vi "Config - Fire CMD.vi"(8 "error in (no error)":errorcluster, 10 "Config CMD":T1, 11 "View Model":T2) -> (0 "error out":errorcluster, 3 "View Model":T2)   [LabVIEW 2017]
doc: "Generates User Event for Configuration command."
uses:
  View Model/Controls/View Model.ctl
  Error Handler/Controls/Error Model.ctl
  Error Handler/Controls/Error Data.ctl
  Error Handler/Controls/Error Type.ctl
  View Model/Controls/Shared Model.ctl
  Controls/Config Model.ctl
  Controls/Config CMD.ctl
  Controls/Config Data.ctl
  ATM Controller/Controls/Controller Model.ctl
  ATM Controller/Controls/Controller Overhead.ctl
  ATM Controller/Controls/Controller States.ctl
  ATM Controller/Controls/Controller Message Data.ctl
  ATM Controller/Controls/Controller Message Name.ctl
  Views/User Console View/Controls/User Console - Keypad.ctl
  Views/User Console View/Controls/User Console - Transactions.ctl
  ATM Controller/Controls/Controller CMD.ctl
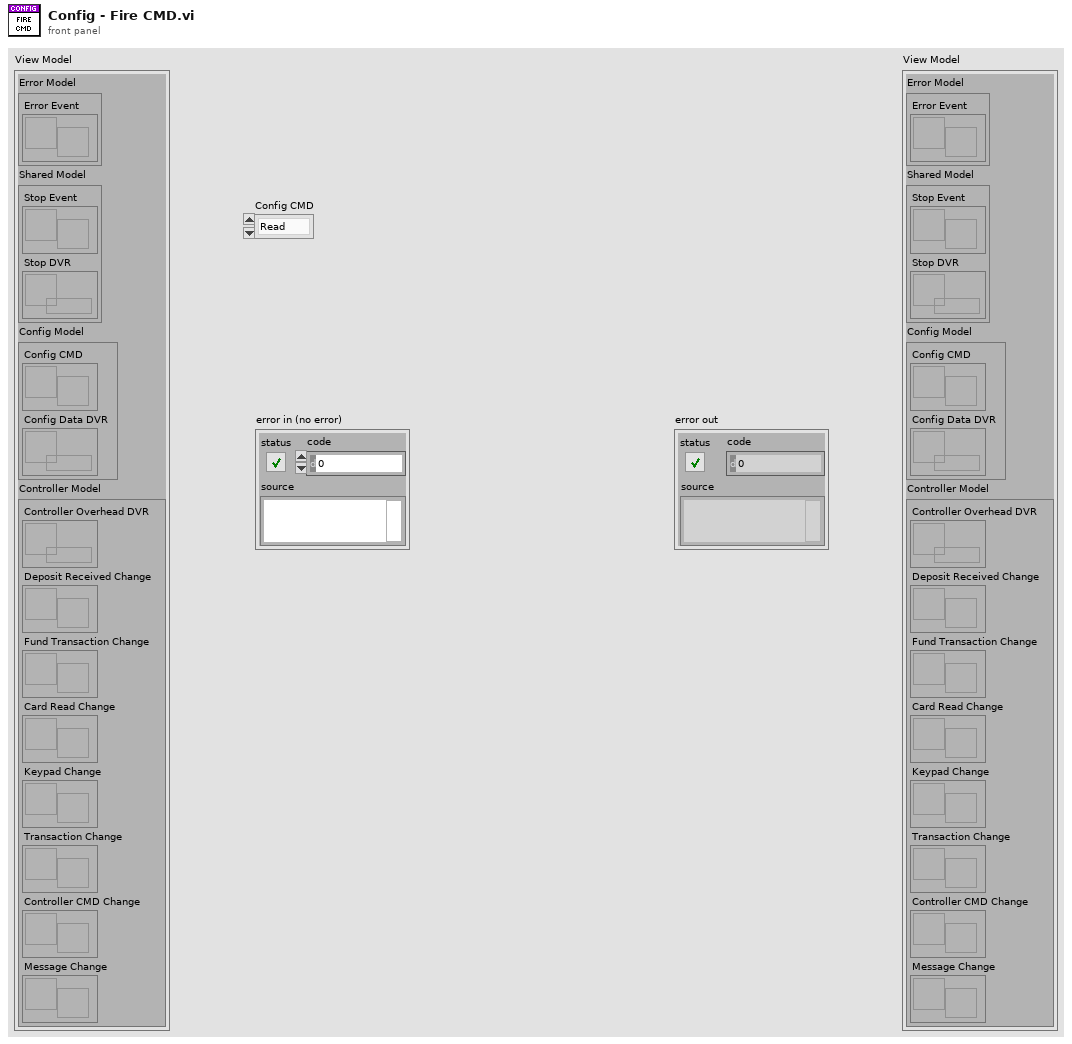
[diagram p1: front panel]
types:
  T1 = typedef "Config CMD.ctl" = enum16{"Read", "Update", "Search"}
  T2 = typedef "View Model.ctl" = cluster{"Error Model":T3, "Shared Model":T4, "Config Model":T5, "Controller Model":T6}
  T3 = typedef "Error Model.ctl" = cluster{"Error Event":refnum<user-event>}
  T4 = typedef "Shared Model.ctl" = cluster{"Stop Event":refnum<user-event>, "Stop DVR":refnum<data-value>}
  T5 = typedef "Config Model.ctl" = cluster{"Config CMD":refnum<user-event>, "Config Data DVR":refnum<data-value>}
  T6 = typedef "Controller Model.ctl" = cluster{"Controller Overhead DVR":refnum<data-value>, "Deposit Received Change":refnum<user-event>, "Fund Transaction Change":refnum<user-event>, "Card Read Change":refnum<user-event>, "Keypad Change":refnum<user-event>, "Transaction Change":refnum<user-event>, "Controller CMD Change":refnum<user-event>, "Message Change":refnum<user-event>}
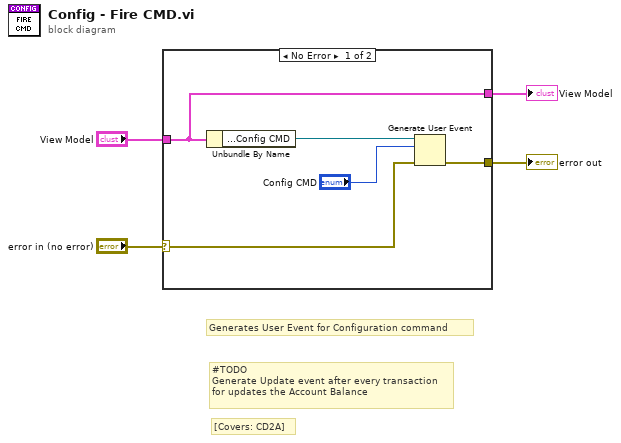
[diagram p0: block diagram]
diagram:
  # "[Covers: CD2A]"
  # "#TODO\nGenerate Update event after every transaction\nfor updates the Account Balance"
  # "Generates User Event for Configuration command"
  n1 = case shown="No Error" "error in (no error)" {
    selector: "error in (no error)" -> [w7 w10]
    tunnel: "View Model" -> [w6 w11]
    tunnel: [w6 w11] -> w2
    tunnel: [w5 w10] -> w1
    frame No Error {
      n2 = Unbundle By Name(w6) -> ("Config Model.Config CMD"=w9:refnum<user-event>)
      n3 = Generate User Event(user event=w9, event data cluster="Config CMD", error in=w7) -> (error out=w5:errorcluster)  [unwired: 1 in, 1 out]
    }
    frame Error {
    }
  }
  "View Model" <- w2
  "error out" <- w1
